vi "Framework Source Test.vi"() -> ()   [LabVIEW 2017]
uses:
  DSF Configuration API/Public/Controls/DSF Engine Framework Configuration.ctl
  DSF Configuration API/Public/Controls/DSF Engine Plugin Configuration.ctl
  DSF Configuration API/Public/Controls/DSF Timing Info.ctl
  DSF Configuration API/Public/Controls/DSF Engine Plugin Thread Configuration.ctl
  DSF Configuration API/Public/Controls/DSF Settings Info.ctl
  DSF Configuration API/Public/Controls/DSF Engine Transfer Group Configuration.ctl
  DSF Configuration API/Public/Controls/DSF Direction.ctl
  DSF Configuration API/Public/Controls/DSF Engine Transfer Configuration.ctl
  DSF Configuration API/Public/Controls/DSF Byte Order.ctl
  DSF Configuration API/Public/Controls/DSF Engine Channel Configuration.ctl
  DSF Configuration API/Public/Controls/DSF Data Type.ctl
  DSF Configuration API/Public/Controls/DSF Timeout Behavior.ctl
  Classes/Framework/Framework Options.ctl
  Typedefs/FIFO Flags.ctl
  Classes/Thread/Thread Options.ctl
  Typedefs/Plugin Flags.ctl
  Typedefs/Performance Options.ctl
  Classes/Framework/Framework.lvclass
  <vilib>/NI/Memory Manager/Classes/Pointer/Pointer.lvclass/Pointer.ctl
  Classes/Framework/Framework.lvclass/Framework.ctl
  Classes/Status/Performance.lvclass/Performance.ctl
  Classes/Plugin/Plugin.lvclass/Plugin.ctl
  Classes/Timing/Timing.lvclass/Timing.ctl
  Classes/Transfer Group/Transfer Group.lvclass/Transfer Group.ctl
  <vilib>/NI/Memory Manager/Classes/Pointer/Set Address.vi
  <vilib>/NI/Memory Manager/Classes/Pointer/Set Size.vi
  <vilib>/NI/Memory Manager/Classes/Pointer/Set Internal.vi
  Classes/Plugin/Is Active.vi
  Classes/Plugin/Set Active.vi
  Classes/Plugin/Active Transfer Groups.vi
  Classes/Plugin/Increment Iteration.vi
  <vilib>/NI/Memory Manager/Classes/Pointer/Get Internal.vi
  <vilib>/NI/Memory Manager/Classes/Pointer/Errors.vi
  <vilib>/NI/Memory Manager/Classes/Pointer/Zone.vi
  <vilib>/NI/Memory Manager/Classes/Pointer/Check Null Pointer.vi
  Classes/Status/Write Period.vi
  Classes/Timing/Is Active Cycle.vi
  Classes/Transfer Group/Is Active.vi
  Classes/Transfer Group/Set Active.vi
  Classes/Plugin/Iteration.vi
  Classes/Timing/Increment Iteration.vi
  <vilib>/NI/Memory Manager/Classes/Pointer/Create Error.vi
  <vilib>/NI/Memory Manager/Classes/Pointer/Null Pointer.vi
  <vilib>/NI/Memory Manager/Classes/Pointer/Is Null.vi
  <vilib>/NI/Memory Manager/Classes/Pointer/Write.vi
  <vilib>/NI/Memory Manager/Classes/Pointer/Write U32.vi
  Classes/Timing/Get Decimation.vi
  Classes/Timing/Get Offset.vi
  Classes/Plugin/Get Timing.vi
  Classes/Timing/Get Iteration.vi
  <vilib>/NI/Memory Manager/VIs/New Error Cluster Constant.vi
  <vilib>/NI/Memory Manager/VIs/New Error Cluster Constant (512B).vi
  <vilib>/NI/Memory Manager/VIs/Error Cluster.Set Status.vi
  <vilib>/NI/Memory Manager/VIs/Error Cluster.Set Code.vi
  <vilib>/NI/Memory Manager/VIs/Error Cluster.Set VI Source.vi
  <vilib>/NI/Memory Manager/Constants/Constants.vi
  <vilib>/NI/Memory Manager/Constants/Library Name.vi
  <vilib>/NI/Memory Manager/Classes/Pointer/Pointer Error Info.vi
  <vilib>/NI/Memory Manager/VIs/Source.Write.String.vi
  <vilib>/NI/Memory Manager/Constants/Pointer Class Name.vi
  <vilib>/NI/Memory Manager/Classes/Pointer/Write (No Check).vi
  <vilib>/NI/Memory Manager/Classes/Pointer/Write (No Check) U32.vi
  <vilib>/NI/Memory Manager/Classes/Pointer/Check Move.vi
  <vilib>/NI/Memory Manager/Classes/Pointer/Check Count.vi
  <vilib>/NI/Memory Manager/Classes/Pointer/Check Bounds (Power of 2).vi
  <vilib>/NI/Memory Manager/Classes/Pointer/Out of Bounds.vi
  <vilib>/NI/Memory Manager/Classes/Pointer/Check Bounds.vi
  <vilib>/NI/Memory Manager/Classes/Pointer/Write Pointer Size.vi
  <vilib>/NI/Memory Manager/VIs/Source.Write.Scalar.Base10.vi
  <vilib>/NI/Memory Manager/VIs/Source.Write.Scalar.Base10 (U64).vi
  <vilib>/NI/Memory Manager/Classes/Pointer/Check Pointer Bounds.vi
  <vilib>/NI/Memory Manager/Classes/Pointer/Check Buffer Bounds.vi
  <vilib>/NI/Memory Manager/Classes/Pointer/Buffer Underflow.vi
  <vilib>/NI/Memory Manager/Classes/Pointer/Pointer.lvclass
  DSF Configuration API/Configuration Session.lvclass
  DSF Core.lvlib
  Classes/Status/Performance.lvclass
panel:
  in  "dsf configuration file path":path=path "C:/Users/Admin/Desktop/test2.dsf"
  out "iteration":u64
  out "error out":errorcluster
  in  "options":T1={"FIFO Options"={"Infinite Timeouts"=TRUE}, "Thread Options"={"Show FP On Call"=TRUE, "Close FP After Call"=TRUE, "Allow Debugging"=TRUE, "Show Menu Bar"=TRUE, "Reposition Windows"=TRUE}, "Plugin Options"={"Default Components"=TRUE}, "Performance Options"={"Measure Period"=FALSE, "Measure Rx/Tx Duration"=FALSE}}
  in  "framework configuration":T6={"components directory"=path "C:/Builds/Data Sharing Framework/Windows/32/Components", "Plugins"=[{"name"="UDP", "components"=["UDP"], "cycle timing"={"priority"=100, "decimation"=2, "offset"=0}, "threads"=[{"buffer converter settings"=[], "transceiver settings"=[{"key"="Local Port", "value"="50000"}], "processor"=-2, "priority offset"=-2}, {"buffer converter settings"=[], "transceiver settings"=[{"key"="Local Port", "value"="50001"}], "processor"=-2, "priority offset"=-2}, {"buffer converter settings"=[], "transceiver settings"=[{"key"="Local Port", "value"="50002"}], "processor"=-2, "priority offset"=-2}, {"buffer converter settings"=[], "transceiver settings"=[{"key"="Local Port", "value"="50003"}], "processor"=-2, "priority offset"=-2}], "Transfer Groups"=[{"name"="Group0", "direction"=enum."Tx", "cycle timing"={"priority"=100, "decimation"=5, "offset"=0}, "thread index"=0, "settings"=[], "Transfers"=[{"name"="Transfer0", "byte order"=enum."big-endian", "settings"=[{"key"="Destination Port", "value"="60000"}, {"key"="Destination Address", "value"="localhost"}], "channels"=[{"string offset"=0, "string data type"=enum."SGL", "engine data type"=enum."DBL", "name"="Temp", "settings"=[]}, {"string offset"=4, "string data type"=enum."DBL", "engine data type"=enum."DBL", "name"="RPM", "settings"=[]}, {"string offset"=12, "string data type"=enum."Bool", "engine data type"=enum."DBL", "name"="LED", "settings"=[]}, {"string offset"=13, "string data type"=enum."I32", "engine data type"=enum."DBL", "name"="Count", "settings"=[]}]}], "timeout behavior"=enum."Increment Late Count"}], "settings"=[]}]}
  in  "stop":bool
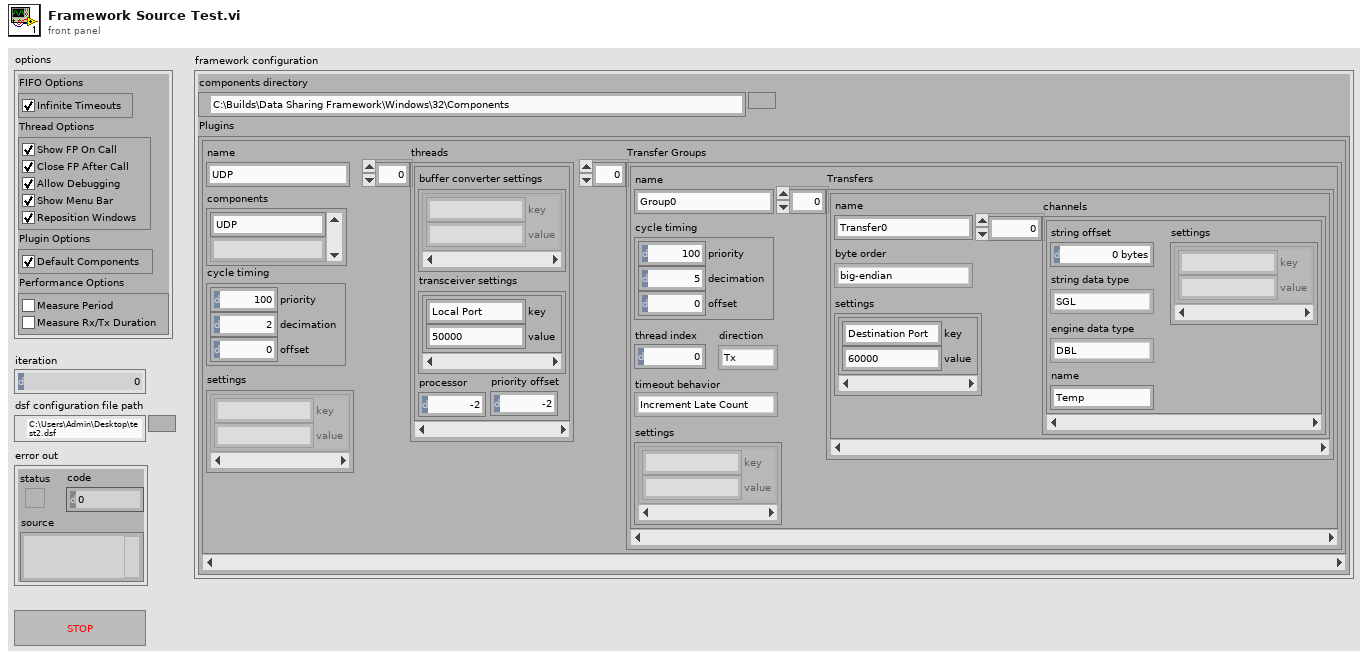
[diagram p1: front panel]
types:
  T1 = typedef "DSF Core.lvlib/Framework.lvclass/Framework Options.ctl" = cluster{"FIFO Options":T2, "Thread Options":T3, "Plugin Options":T4, "Performance Options":T5}
  T2 = typedef "DSF Core.lvlib/FIFO Flags.ctl" = cluster{"Infinite Timeouts":bool}
  T3 = typedef "DSF Core.lvlib/Thread Options.ctl" = cluster{"Show FP On Call":bool, "Close FP After Call":bool, "Allow Debugging":bool, "Show Menu Bar":bool, "Reposition Windows":bool}
  T4 = typedef "DSF Core.lvlib/Plugin Flags.ctl" = cluster{"Default Components":bool}
  T5 = typedef "DSF Core.lvlib/Performance.lvclass/Performance Options.ctl" = cluster{"Measure Period":bool, "Measure Rx/Tx Duration":bool}
  T6 = typedef "DSF Core.lvlib/DSF Engine Framework Configuration.ctl" = cluster{"components directory":path, "Plugins":T7[]}
  T7 = typedef "DSF Core.lvlib/DSF Engine Plugin Configuration.ctl" = cluster{"name":string, "components":string[], "cycle timing":T8, "threads":T9[], "Transfer Groups":T11[], "settings":T10}
  T8 = typedef "DSF Core.lvlib/DSF Timing Info.ctl" = cluster{"priority":u64, "decimation":u64, "offset":u64}
  T9 = typedef "DSF Core.lvlib/DSF Engine Plugin Thread Configuration.ctl" = cluster{"buffer converter settings":T10, "transceiver settings":T10, "processor":i32, "priority offset":i16}
  T10 = typedef "DSF Core.lvlib/DSF Settings Info.ctl" = cluster{"key":string, "value":string}[]
  T11 = typedef "DSF Core.lvlib/DSF Engine Transfer Group Configuration.ctl" = cluster{"name":string, "direction":T12, "cycle timing":T8, "thread index":i32, "settings":T10, "Transfers":T13[], "timeout behavior":T17}
  T12 = typedef "DSF Core.lvlib/DSF Direction.ctl" = enum8{"Tx", "Rx"}
  T13 = typedef "DSF Core.lvlib/DSF Engine Transfer Configuration.ctl" = cluster{"name":string, "byte order":T14, "settings":T10, "channels":T15[]}
  T14 = typedef "DSF Core.lvlib/DSF Byte Order.ctl" = enum8{"big-endian", "little-endian"}
  T15 = typedef "DSF Core.lvlib/DSF Engine Channel Configuration.ctl" = cluster{"string offset":u64, "string data type":T16, "engine data type":T16, "name":string, "settings":T10}
  T16 = typedef "DSF Core.lvlib/DSF Data Type.ctl" = enum8{"Bool", "SGL", "DBL", "I8", "I16", "I32", "I64", "U8", "U16", "U32", "U64"}
  T17 = typedef "DSF Core.lvlib/DSF Timeout Behavior.ctl" = enum8{"Increment Late Count", "Throw Error"}
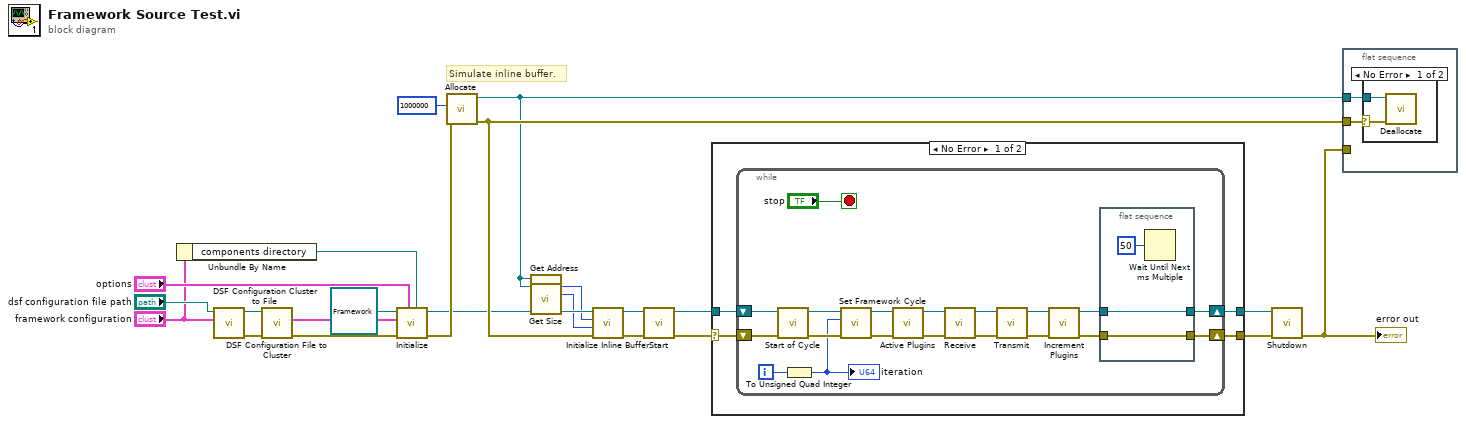
[diagram p0: block diagram]
diagram:
  # "Simulate inline buffer."
  n1 = Unbundle By Name("framework configuration") -> ("components directory"=w10:path)
  n2 = call "DSF Configuration Cluster to File.vi"("framework configuration"="framework configuration", "dsf configuration file path"="dsf configuration file path") -> ("error out"=w14:errorcluster, "dsf configuration file path dup"=w11:path)  [unwired: 8 in]
  n3 = call "DSF Configuration File to Cluster.vi"("error in (no error)"=w14, "dsf configuration file path"=w11) -> ("error out"=w13:errorcluster, "framework configuration out"=w1:T6)  [unwired: 7 in, 1 out]
  n4 = call-dynamic "Initialize.vi"("components directory"=w10, "options"="options", "error in (no error)"=w13, "framework configuration"=w1, "Framework in"=refnum<class "Framework.lvclass"> refnum) -> ("error out"=w9:errorcluster, "Framework out"=w8:refnum<class "Framework.lvclass">)  [unwired: 5 in]
  n5 = call <vilib>:"Allocate.vi"("error in (no error)"=w9, "size"=u64 1000000) -> ("error out"=w18:errorcluster, "Pointer out"=w15:refnum<class "Pointer.lvclass">)  [unwired: 8 in]
  n6 = call <vilib>:"Get Address.vi"("Pointer in"=w15) -> ("address"=w6:u64)  [unwired: 9 in, 1 out]
  n7 = call <vilib>:"Get Size.vi"("Pointer in"=w15) -> ("size"=w7:u64)  [unwired: 9 in, 1 out]
  n8 = call "Initialize Inline Buffer.vi"("error in (no error)"=w18, "size"=w7, "address"=w6, "Framework in"=w8) -> ("error out"=w3:errorcluster, "Framework out"=w4:refnum<class "Framework.lvclass">)  [unwired: 6 in]
  n9 = call-dynamic "Start.vi"("error in (no error)"=w3, "Framework in"=w4) -> ("error out"=w16:errorcluster, "Framework out"=w17:refnum<class "Framework.lvclass">)  [unwired: 8 in]
  n10 = case shown="No Error" w16 {
    selector: w16 -> [w26 w50]
    tunnel: [w24 w50] -> w23
    tunnel: w17 -> [w27 w51]
    tunnel: [w25 w51] -> w22
    frame No Error {
      n11 = while {
        shift-right: [w35] -> w25
        shift-left: w27 -> [w33]
        shift-right: [w34] -> w24
        shift-left: w26 -> [w32]
        i -> [w29]
        stop <- "stop" stop-if-true
        n12 = call "Start of Cycle.vi"("error in (no error)"=w32, "Framework in"=w33) -> ("error out"=w31:errorcluster, "Framework out"=w30:refnum<class "Framework.lvclass">)  [unwired: 8 in]
        n13 = To Unsigned Quad Integer(1:w29) -> (0:w28:u64)
        "iteration" <- w28
        n14 = call "Set Framework Cycle.vi"("error in (no error)"=w31, "iteration"=w28, "Framework in"=w30) -> ("error out"=w43:errorcluster, "Framework out"=w44:refnum<class "Framework.lvclass">)  [unwired: 7 in]
        n15 = call "Active Plugins.vi"("error in (no error)"=w43, "Framework in"=w44) -> ("error out"=w41:errorcluster, "Framework out"=w42:refnum<class "Framework.lvclass">)  [unwired: 8 in]
        n16 = call "Receive.vi"("error in (no error)"=w41, "Framework in"=w42) -> ("error out"=w46:errorcluster, "Framework out"=w45:refnum<class "Framework.lvclass">)  [unwired: 8 in]
        n17 = call "Transmit.vi"("error in (no error)"=w46, "Framework in"=w45) -> ("error out"=w39:errorcluster, "Framework out"=w40:refnum<class "Framework.lvclass">)  [unwired: 8 in]
        n18 = call "Increment Plugins.vi"("error in (no error)"=w39, "Framework in"=w40) -> ("error out"=w36:errorcluster, "Framework out"=w37:refnum<class "Framework.lvclass">)  [unwired: 8 in]
        n19 = flat-sequence {
          tunnel: w37 -> [w48]
          tunnel: w36 -> [w47]
          tunnel: [w48] -> w35
          tunnel: [w47] -> w34
          frame #0 {
            n20 = Wait Until Next ms Multiple(millisecond multiple=u32 50 ("milliseconds to wait")) -> ()  [unwired: 1 out]
          }
        }
      }
    }
    frame Error {
    }
  }
  n21 = call-dynamic "Shutdown.vi"("error in (no error)"=w23, "Framework in"=w22) -> ("error out"=w19:errorcluster)  [unwired: 8 in, 1 out]
  "error out" <- w19
  n22 = flat-sequence {
    tunnel: w15 -> [w53]
    tunnel: w19 -> [_]
    tunnel: w18 -> [w52]
    frame #0 {
      n23 = case shown="No Error" w52 {
        selector: w52 -> [w54 _]
        tunnel: w53 -> [w55 _]
        frame No Error {
          n24 = call <vilib>:"Deallocate.vi"("error in (no error)"=w54, "Pointer in"=w55) -> ()  [unwired: 8 in, 2 out]
        }
        frame Error {
        }
      }
    }
  }
